vi "Find Parse State Queue from While Loop.vi"(8 "error in (no error)":errorcluster, 11 "WhileLoop in":refnum<vi>) -> (0 "error out":errorcluster, 1 "CaseStructure":refnum<vi>, 2 "Parse State Queue":refnum<vi>)   [LabVIEW 2013, in "JKI State Machine API.lvlib" / "JKI SM.lvclass"]
uses:
  JKI SM.lvclass
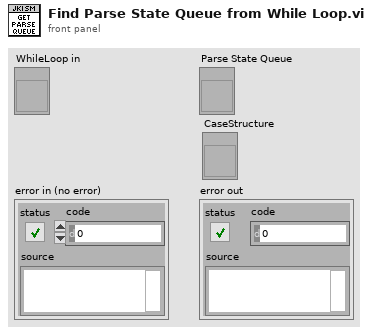
[diagram p1: front panel]
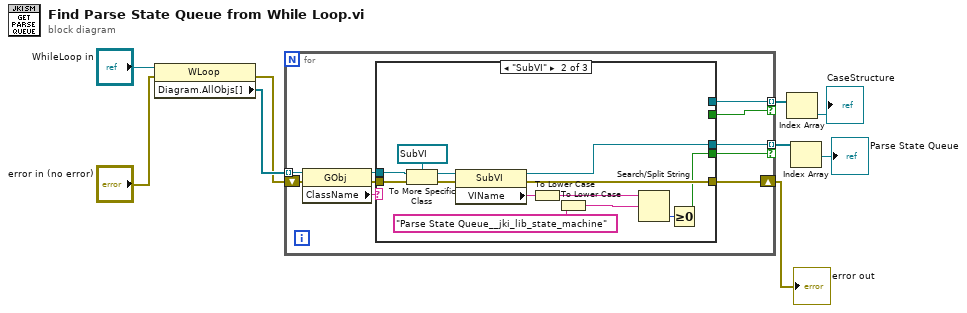
[diagram p0: block diagram]
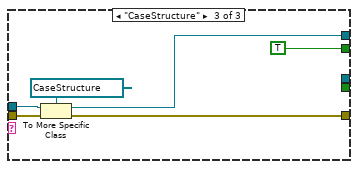
[diagram p3: hidden frame]
diagram:
  n1 = property class="WLoop"(reference="WhileLoop in", error in="error in (no error)") -> (error out=w6:errorcluster, "Diagram.AllObjs[]"=w9:refnum<vi>[])  [unwired: 1 out]
  n2 = for {
    tunnel: w9 -> [w19] mode=indexing
    shift-right: [w14] -> w5
    shift-left: w6 -> [w15]
    tunnel: [w13] -> w2 mode=indexing if=w10
    tunnel: [w12] -> w4 mode=indexing if=w11
    n3 = property class="GObj"(reference=w19, error in=w15) -> (reference out=w17:refnum<vi>, error out=w16:errorcluster, "ClassName"=w18:string)
    n4 = case shown="\"SubVI\"" w18 {
      tunnel: w17 -> [_ w32 w38]
      tunnel: w16 -> [w20 w31 w37]
      tunnel: [w20 w26 w36] -> w14
      tunnel: [_ w25 _] -> w13
      tunnel: [_ _ w35] -> w12
      tunnel: [_ _ TRUE] -> w11
      tunnel: [_ w21 _] -> w10
      frame Default {
      }
      frame "SubVI" {
        n5 = To More Specific Class(target class=refnum<vi> refnum ("SubVI Refnum"), reference=w32, error in=w31) -> (specific class reference=w30:refnum<vi>, error out=w29:errorcluster)
        n6 = property class="SubVI"(reference=w30, error in=w29) -> (reference out=w25:refnum<vi>, error out=w26:errorcluster, "VIName"=w28:string)
        n7 = To Lower Case(string=w28) -> (all lower case string=w23:string)
        n8 = To Lower Case(string="Parse State Queue__jki_lib_state_machine" ("VI Name")) -> (all lower case string=w24:string)
        n9 = Search/Split String(string=w23, search string/char (-)=w24) -> (offset of match=w22:i32)  [unwired: 1 in, 2 out]
        n10 = Greater Or Equal To 0?(x=w22) -> (x >= 0?=w21:bool)
      }
      frame "CaseStructure" {
        n11 = To More Specific Class(target class=refnum<vi> refnum ("CaseSel Refnum"), reference=w38, error in=w37) -> (specific class reference=w35:refnum<vi>, error out=w36:errorcluster)
      }
    }
  }
  "error out" <- w5
  n12 = Index Array(array=w4) -> (element=→"CaseStructure":refnum<vi>)  [unwired: 1 in]
  n13 = Index Array(array=w2) -> (element=→"Parse State Queue":refnum<vi>)  [unwired: 1 in]
